vi "Create Bucket Storage Policy.vi"(8 "error in (no error)":errorcluster, 10 "Role Name":string, 11 "Bucket in":refnum<class "Bucket.lvclass">) -> (0 "error out":errorcluster, 3 "Bucket out":refnum<class "Bucket.lvclass">)   [LabVIEW 2015, in "NI_AWS_S3.lvlib" / "Bucket.lvclass"]
uses:
  Bucket.lvclass
  Bucket.lvclass/Bucket.ctl
  Core/HTTP Request/HTTP Request.lvclass/HTTP Request.ctl
  Read Name.vi
  Core/HTTP Request/Read Credentials.vi
  IAM/IAM Session/IAM Session.lvclass
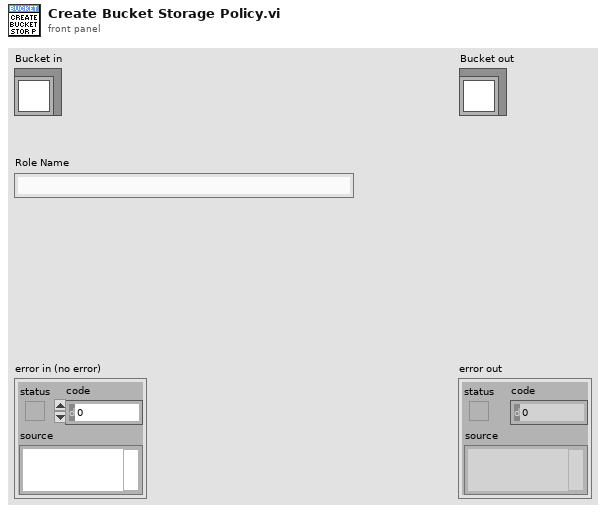
[diagram p1: front panel]
types:
  T1 = typedef "NI_AWS_Core.lvlib/HTTP Request.lvclass/AWS Credentials.ctl" = cluster{"Access Key":string, "Secret Key":string}
  T2 = typedef "NI_AWS_IAM.lvlib/Policy.ctl" = cluster{"Name":string, "Default Version ID":string, "ID":string, "Path":string, "ARN":string, "Attachment Count":i32, "Creation Date":string, "Last Updated Date":string}
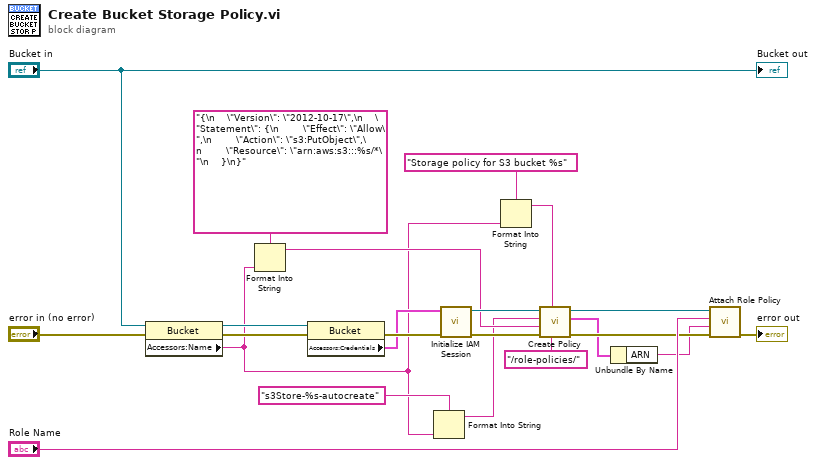
[diagram p0: block diagram]
diagram:
  n1 = property class="Bucket"(reference="Bucket in", error in="error in (no error)") -> (reference out=w3:refnum<class "Bucket.lvclass">, error out=w5:errorcluster, "Accessors:Name"=w2:string)
  n2 = Format Into String(format string="{\n    \"Version\": \"2012-10-17\",\n    \"Statement\": {\n        \"Effect\": \"Allow\",\n        \"Action\": \"s3:PutObject\",\n        \"Resource\": \"arn:aws:s3:::%s/*\"\n    }\n}", w2) -> (resulting string=w8:string)  [unwired: 2 in, 1 out]
  n3 = property class="Bucket"(reference=w3, error in=w5) -> (error out=w20:errorcluster, "Accessors:Credentials"=w19:T1)  [unwired: 1 out]
  n4 = Format Into String(format string="s3Store-%s-autocreate", w2) -> (resulting string=w6:string)  [unwired: 2 in, 1 out]
  n5 = call "Initialize IAM Session.vi"("error in (no error)"=w20, "AWS Credentials"=w19) -> ("error out"=w18:errorcluster, "IAM Session"=w17:refnum<class "IAM Session.lvclass">)  [unwired: 8 in]
  n6 = Format Into String(format string="Storage policy for S3 bucket %s", w2) -> (resulting string=w13:string)  [unwired: 2 in, 1 out]
  n7 = call "Create Policy.vi"("Path"="/role-policies/", "Description"=w13, "error in (no error)"=w18, "Document"=w8, "Name"=w6, "IAM Session in"=w17) -> ("error out"=w16:errorcluster, "Created Policy"=w11:T2, "IAM Session out"=w15:refnum<class "IAM Session.lvclass">)  [unwired: 3 in]
  n8 = Unbundle By Name(w11) -> ("ARN"=w10:string)
  n9 = call "Attach Role Policy.vi"("error in (no error)"=w16, "Policy ARN"=w10, "Role Name"="Role Name", "IAM Session in"=w15) -> ("error out"=→"error out":errorcluster)  [unwired: 6 in, 1 out]
  "Bucket out" <- "Bucket in"
